vi "Initialize.vi"(8 "error in (no error)":errorcluster, 11 "Instruments in":refnum<class "Instruments.lvclass">) -> (0 "error out":errorcluster, 3 "Instruments out":refnum<class "Instruments.lvclass">)   [LabVIEW 2023, in "Instruments.lvlib" / "Instruments.lvclass"]
doc: "This is an abstraction that is already implemented in the pre-launch init routine\n\nInitialize is called <b>after</b> the event reference queues and caller and self enqueuers are created. \n\nBe sure to inspect the parent method to determine whether or not call parent method is required."
uses:
  Library/Instruments.lvclass
  builds/Framework/Configuration.lvlibp/Library/Configuration.lvclass
  builds/Framework/Engine.lvlibp/Engine/Library/Engine.lvclass
  C:/Users/Public/Documents/Development/builds/Framework/Engine.lvlibp/Engine/Library/Engine.lvclass
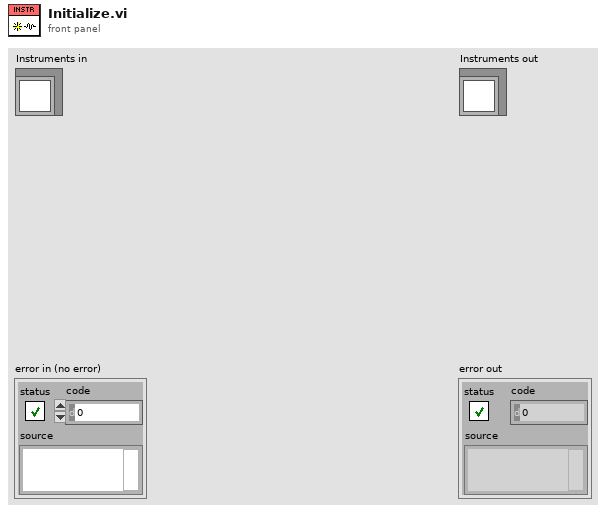
[diagram p1: front panel]
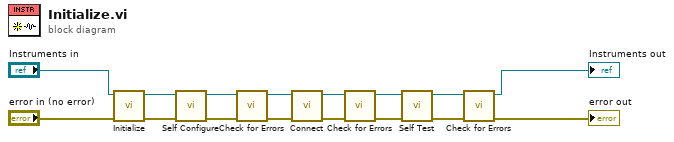
[diagram p0: block diagram]
diagram:
  n1 = call-parent "Initialize.vi"("error in (no error)"="error in (no error)", "Configuration in"="Instruments in") -> ("error out"=w14:errorcluster, "Configuration out"=w13:refnum<class "Instruments.lvclass">)  [unwired: 8 in]
  n2 = call-dynamic "Self Configure.vi"("error in (no error)"=w14, "Instruments in"=w13) -> ("error out"=w11:errorcluster, "Instruments out"=w12:refnum<class "Instruments.lvclass">)  [unwired: 8 in]
  n3 = call "Check for Errors.vi"("error in"=w11, "Engine in"=w12) -> ("error out"=w9:errorcluster, "Engine out"=w10:refnum<class "Instruments.lvclass">)  [unwired: 8 in]
  n4 = call-dynamic "Connect.vi"("error in (no error)"=w9, "Instruments in"=w10) -> ("error out"=w8:errorcluster, "Instruments out"=w7:refnum<class "Instruments.lvclass">)  [unwired: 8 in]
  n5 = call "Check for Errors.vi"("error in"=w8, "Engine in"=w7) -> ("error out"=w6:errorcluster, "Engine out"=w5:refnum<class "Instruments.lvclass">)  [unwired: 8 in]
  n6 = call-dynamic "Self Test.vi"("error in (no error)"=w6, "Instruments in"=w5) -> ("error out"=w4:errorcluster, "Instruments out"=w3:refnum<class "Instruments.lvclass">)  [unwired: 8 in]
  n7 = call "Check for Errors.vi"("error in"=w4, "Engine in"=w3) -> ("error out"=→"error out":errorcluster, "Engine out"=→"Instruments out":refnum<class "Instruments.lvclass">)  [unwired: 8 in]
